vi "test_wire.vi"() -> ()   [LabVIEW 2023]
uses:
  BlockDiagram/BlockDiagram.lvclass
  C:/projects/TLC_Scripto/Source/AbstractDiagram/AbstractDiagram.lvclass
  AbstractDiagram/Read wires.vi
  Wire/Read wireRef.vi
  Wire/Wire.lvclass
  TLC_Scripto.lvlib
  AbstractDiagram/AbstractDiagram.lvclass
  Structure/Structure.lvclass
  C:/projects/TLC_Scripto/Source/GObject/GObject.lvclass
  C:/projects/TLC_Scripto/Source/Generic/Generic.lvclass
  C:/projects/TLC_Scripto/Source/BlockDiagram/BlockDiagram.lvclass
panel:
  out "Joints[]":T1(array[cluster])
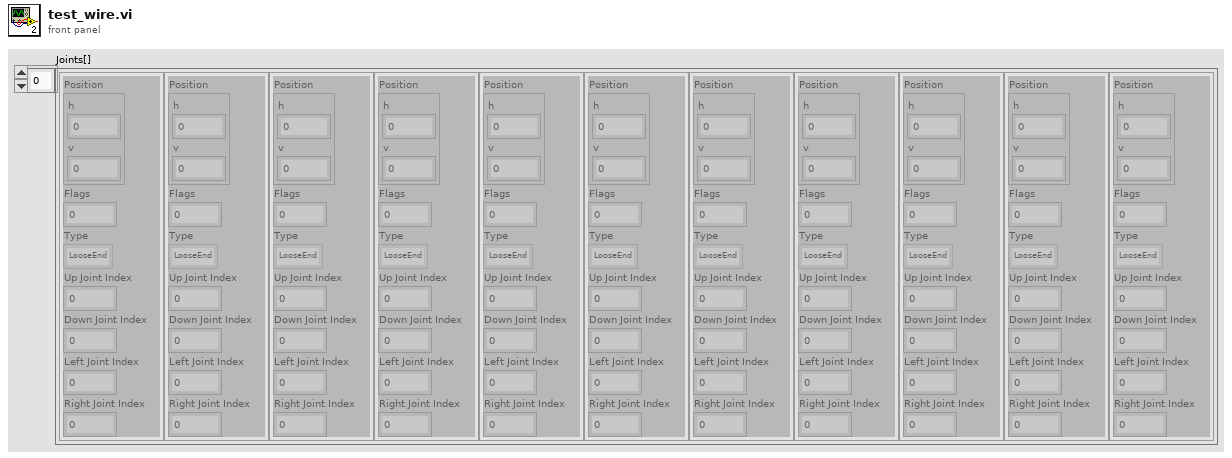
[diagram p1: front panel]
types:
  T1 = cluster{"Position":cluster{"h":i16, "v":i16}, "Flags":i32, "Type":enum32{"LooseEnd", "Endpoint", "Bend", "Junction"}, "Up Joint Index":i16, "Down Joint Index":i16, "Left Joint Index":i16, "Right Joint Index":i16}[]
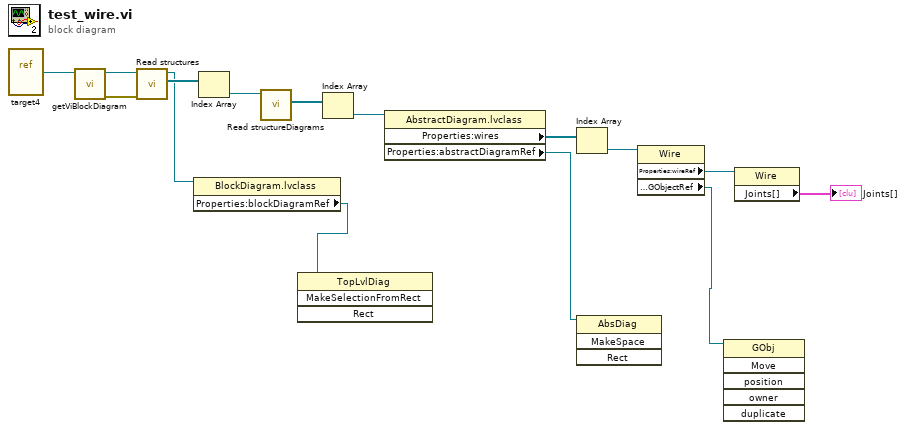
[diagram p0: block diagram]
diagram:
  n1 = vi-ref "target4.vi"() -> (w15:refnum<vi>)
  n2 = call "getViBlockDiagram.vi"("ViRef"=w15) -> ("error out"=w13:errorcluster, "topMostBlockDiagram"=w14:refnum<class "BlockDiagram.lvclass">)  [unwired: 9 in]
  n3 = call "Read structures.vi"("error in (no error)"=w13, "BlockDiagram in"=w14) -> ("structures"=w12:refnum<class "Structure.lvclass">[], "BlockDiagram out"=w2:refnum<class "BlockDiagram.lvclass">)  [unwired: 7 in, 1 out]
  n4 = property class="BlockDiagram.lvclass"(reference=w2) -> ("Properties:blockDiagramRef"=w1:refnum<vi>)  [unwired: 1 in, 2 out]
  n5 = Index Array(array=w12) -> (element=w9:refnum<class "Structure.lvclass">)  [unwired: 1 in]
  n6 = call "Read structureDiagrams.vi"("Structure In"=w9) -> ("strctureDiagrams"=w10:refnum<class "AbstractDiagram.lvclass">[])  [unwired: 8 in, 2 out]
  n7 = invoke class="TopLvlDiag" method="MakeSelectionFromRect"(reference=w1) -> ()  [unwired: 3 in, 4 out]
  n8 = Index Array(array=w10) -> (element=w11:refnum<class "AbstractDiagram.lvclass">)  [unwired: 1 in]
  n9 = property class="AbstractDiagram.lvclass"(reference=w11) -> ("Properties:wires"=w8:refnum<class "Wire.lvclass">[], "Properties:abstractDiagramRef"=w3:refnum<vi>)  [unwired: 1 in, 2 out]
  n10 = Index Array(array=w8) -> (element=w7:refnum<class "Wire.lvclass">)  [unwired: 1 in]
  n11 = invoke class="AbsDiag" method="MakeSpace"(reference=w3) -> ()  [unwired: 3 in, 4 out]
  n12 = property class="Wire"(reference=w7) -> ("Properties:wireRef"=w6:refnum<vi>, "Properties:GObjectRef"=w4:refnum<vi>)  [unwired: 1 in, 2 out]
  n13 = invoke class="GObj" method="Move"(reference=w4) -> ()  [unwired: 5 in, 6 out]
  n14 = property class="Wire"(reference=w6) -> ("Joints[]"=→"Joints[]":T1)  [unwired: 1 in, 2 out]
